vi "Array Notation Name.vi"(8 "error in (no error)":errorcluster, 11 "Config Element in":refnum<class "Config Element.lvclass">) -> (0 "error out":errorcluster, 2 "Array Notation Name":string, 3 "Config Element out":refnum<class "Config Element.lvclass">)   [LabVIEW 2020, in "CDM-Config.lvlib" / "Config Element.lvclass"]
uses:
  Config Element.lvclass
  Config Element.lvclass/Config Element.ctl
  Config Manager/Config Manager.lvclass
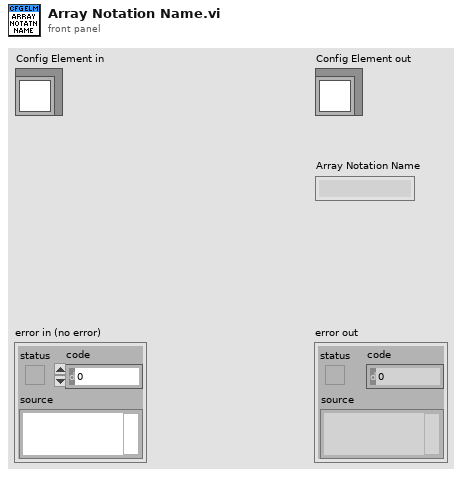
[diagram p1: front panel]
types:
  T1 = typedef "CDM-Config.lvlib/Config Element.lvclass/Ref Data.ctl" = cluster{"Node Info":T2, "Owner":refnum<class>, "Changed":bool, "Name":string, "Value":string, "Meta Data":T3[], "Array":bool}
  T2 = typedef "CDM-Config.lvlib/Node Info.ctl" = cluster{"Index":i32, "Parent":i32, "Children":i32[]}
  T3 = typedef "CDM-Config.lvlib/Meta Data.ctl" = cluster{"Name":string, "Value":string}
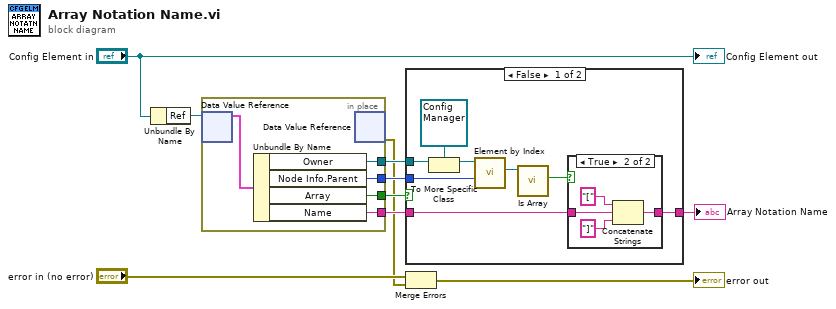
[diagram p0: block diagram]
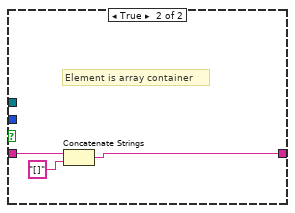
[diagram p3: hidden frame]
diagram:
  n1 = Unbundle By Name("Config Element in") -> ("Ref"=w9:refnum<data-value>)
  n2 = in-place {
    in-place-border: [w14] -> w5
    in-place-border: [w13] -> w6
    in-place-border: [w12] -> w4
    in-place-border: [w11] -> w7
    n3 = in-place-dvr #1(w9) -> (w15:T1)  [unwired: 1 out]
    n4 = Unbundle By Name(w15) -> ("Owner"=w11:refnum<class>, "Node Info.Parent"=w12:i32, "Array"=w13:bool, "Name"=w14:string)
    n5 = in-place-dvr #1() -> (w1:errorcluster)  [unwired: 1 in, 1 out]
  }
  n6 = case shown="False" w6 {
    tunnel: w7 -> [w23 _]
    tunnel: w5 -> [w18 w31]
    tunnel: w4 -> [w20 _]
    tunnel: [w16 w29] -> w3
    frame False {
      n7 = To More Specific Class(target class=refnum<class "Config Manager.lvclass"> refnum ("CDM-Config.lvlib:Config Manager.lvclass"), reference=w23) -> (specific class reference=w21:refnum<class "Config Manager.lvclass">)  [unwired: 1 in, 1 out]
      n8 = call "Element by Index.vi"("Index"=w20, "Config Manager in"=w21) -> ("Element"=w19:refnum<class "Config Element.lvclass">)  [unwired: 7 in, 2 out]
      n9 = call "Is Array.vi"("Config Element in"=w19) -> ("Array"=w17:bool)  [unwired: 8 in, 2 out]
      n10 = case shown="True" w17 {
        tunnel: w18 -> [w24 w28]
        tunnel: [w24 w25] -> w16
        frame False {
        }
        frame True {
          n11 = Concatenate Strings("[" ("string"), w28, "]" ("string")) -> (w25:string)
        }
      }
    }
    frame True {
      # "Element is array container"
      n12 = Concatenate Strings(w31, "[]" ("string")) -> (w29:string)
    }
  }
  "Array Notation Name" <- w3
  n13 = Merge Errors("error in (no error)", w1) -> (→"error out":errorcluster)
  "Config Element out" <- "Config Element in"
